vi "Data Viewer.vi"(6 "menu options":cluster{"open":bool, "save":bool, "view":bool}={"open"=TRUE, "save"=FALSE, "view"=FALSE}, 8 "error in (no error)":errorcluster, 9 "Stop Pointer":refnum<class "Pointer.lvclass">, 10 "Framework Configuration":T1, 11 "DSF":refnum<class "Framework.lvclass">) -> (0 "error out":errorcluster)   [LabVIEW 2017, in "DSF Data Viewer.lvlib"]
uses:
  DSF Data Viewer.lvlib
  Builds/Data Sharing Framework/Current/Core/DSF Core.lvlibp/Engine/Classes/Framework/Framework.lvclass
  Builds/Data Sharing Framework/Current/Core/DSF Core.lvlibp/DSF Configuration API/Public/Controls/DSF Engine Framework Configuration.ctl
  Builds/Data Sharing Framework/Current/Core/DSF Core.lvlibp/DSF Configuration API/Public/Controls/DSF Engine Plugin Configuration.ctl
  Builds/Data Sharing Framework/Current/Core/DSF Core.lvlibp/DSF Configuration API/Public/Controls/DSF Timing Info.ctl
  Builds/Data Sharing Framework/Current/Core/DSF Core.lvlibp/DSF Configuration API/Public/Controls/DSF Engine Plugin Thread Configuration.ctl
  Builds/Data Sharing Framework/Current/Core/DSF Core.lvlibp/DSF Configuration API/Public/Controls/DSF Settings Info.ctl
  Builds/Data Sharing Framework/Current/Core/DSF Core.lvlibp/DSF Configuration API/Public/Controls/DSF Engine Transfer Group Configuration.ctl
  Builds/Data Sharing Framework/Current/Core/DSF Core.lvlibp/DSF Configuration API/Public/Controls/DSF Direction.ctl
  Builds/Data Sharing Framework/Current/Core/DSF Core.lvlibp/DSF Configuration API/Public/Controls/DSF Engine Transfer Configuration.ctl
  Builds/Data Sharing Framework/Current/Core/DSF Core.lvlibp/DSF Configuration API/Public/Controls/DSF Byte Order.ctl
  Builds/Data Sharing Framework/Current/Core/DSF Core.lvlibp/DSF Configuration API/Public/Controls/DSF Engine Channel Configuration.ctl
  Builds/Data Sharing Framework/Current/Core/DSF Core.lvlibp/DSF Configuration API/Public/Controls/DSF Data Type.ctl
  Builds/Data Sharing Framework/Current/Core/DSF Core.lvlibp/DSF Configuration API/Public/Controls/DSF Timeout Behavior.ctl
  <vilib>/NI/Memory Manager/Classes/Pointer/Pointer.lvclass
  <vilib>/NI/Memory Manager/Classes/Pointer/Pointer.lvclass/Pointer.ctl
  Source/Main VI/Application Data.ctl
  Source/Buffer Reader/Buffer Data.ctl
  Builds/Data Sharing Framework/Current/Core/DSF Core.lvlibp/Engine/Classes/Buffer/Buffer.lvclass
  Builds/Data Sharing Framework/Current/Core/DSF Core.lvlibp/Engine/Classes/Transfer Group Status/Transfer Group Status.lvclass
  <vilib>/NI/Memory Manager/Classes/Pointer/Read Bool.vi
  <vilib>/NI/Memory Manager/Classes/Pointer/Write Bool.vi
  <vilib>/NI/Memory Manager/Classes/Pointer/Read (No Check).vi
  <vilib>/NI/Memory Manager/Classes/Pointer/Read (No Check) Bool.vi
  <vilib>/NI/Memory Manager/Classes/Pointer/Check Move.vi
  <vilib>/NI/Memory Manager/Classes/Pointer/Write (No Check).vi
  <vilib>/NI/Memory Manager/Classes/Pointer/Write (No Check) Bool.vi
  <vilib>/NI/Memory Manager/Classes/Pointer/Get Address.vi
  <vilib>/NI/Memory Manager/Classes/Pointer/Set Address.vi
  <vilib>/NI/Memory Manager/Classes/Pointer/Set Size.vi
  <vilib>/NI/Memory Manager/Classes/Pointer/Set Internal.vi
  <vilib>/NI/Memory Manager/Classes/Pointer/Check Null Pointer.vi
  <vilib>/NI/Memory Manager/Classes/Pointer/Check Count.vi
  <vilib>/NI/Memory Manager/Classes/Pointer/Check Bounds (Power of 2).vi
  <vilib>/NI/Memory Manager/Classes/Pointer/Errors.vi
  <vilib>/NI/Memory Manager/Classes/Pointer/Null Pointer.vi
  <vilib>/NI/Memory Manager/Classes/Pointer/Get Size.vi
  <vilib>/NI/Memory Manager/Classes/Pointer/Out of Bounds.vi
  <vilib>/NI/Memory Manager/Classes/Pointer/Check Bounds.vi
  <vilib>/NI/Memory Manager/Classes/Pointer/Create Error.vi
  <vilib>/NI/Memory Manager/VIs/Source.Write.String.vi
  <vilib>/NI/Memory Manager/Classes/Pointer/Write Pointer Size.vi
  <vilib>/NI/Memory Manager/VIs/Source.Write.Scalar.Base10.vi
  <vilib>/NI/Memory Manager/VIs/Source.Write.Scalar.Base10 (U64).vi
  <vilib>/NI/Memory Manager/Classes/Pointer/Check Pointer Bounds.vi
  <vilib>/NI/Memory Manager/Classes/Pointer/Check Buffer Bounds.vi
  <vilib>/NI/Memory Manager/VIs/New Error Cluster Constant.vi
  <vilib>/NI/Memory Manager/VIs/New Error Cluster Constant (512B).vi
  <vilib>/NI/Memory Manager/VIs/Error Cluster.Set Status.vi
  <vilib>/NI/Memory Manager/VIs/Error Cluster.Set Code.vi
  <vilib>/NI/Memory Manager/VIs/Error Cluster.Set VI Source.vi
  <vilib>/NI/Memory Manager/Constants/Constants.vi
  <vilib>/NI/Memory Manager/Constants/Library Name.vi
  <vilib>/NI/Memory Manager/Classes/Pointer/Pointer Error Info.vi
  <vilib>/NI/Memory Manager/Constants/Pointer Class Name.vi
  <vilib>/NI/Memory Manager/Classes/Pointer/Buffer Underflow.vi
  Builds/Data Sharing Framework/Current/Core/DSF Core.lvlibp/DSF Configuration API/Public/Largest Buffer Size (Framework).vi
  Builds/Data Sharing Framework/Current/Core/DSF Core.lvlibp
  Builds/Data Sharing Framework/Current/Core/DSF Core.lvlibp/Engine/Classes/Status/Performance.lvclass
panel:
  in  "Item Tree":string(tree)
  out "Late Count":u64
  out "Iteration":u64
  out "Frequency":dbl format="%.1fHz"
  out "Size":u64 format="%#_3pB"
  out "Null":bool
  out "Decimation":u64
  out "Throughput":dbl format="%#_3pBps"
  out "Buffer":string
  # "Data Viewer"
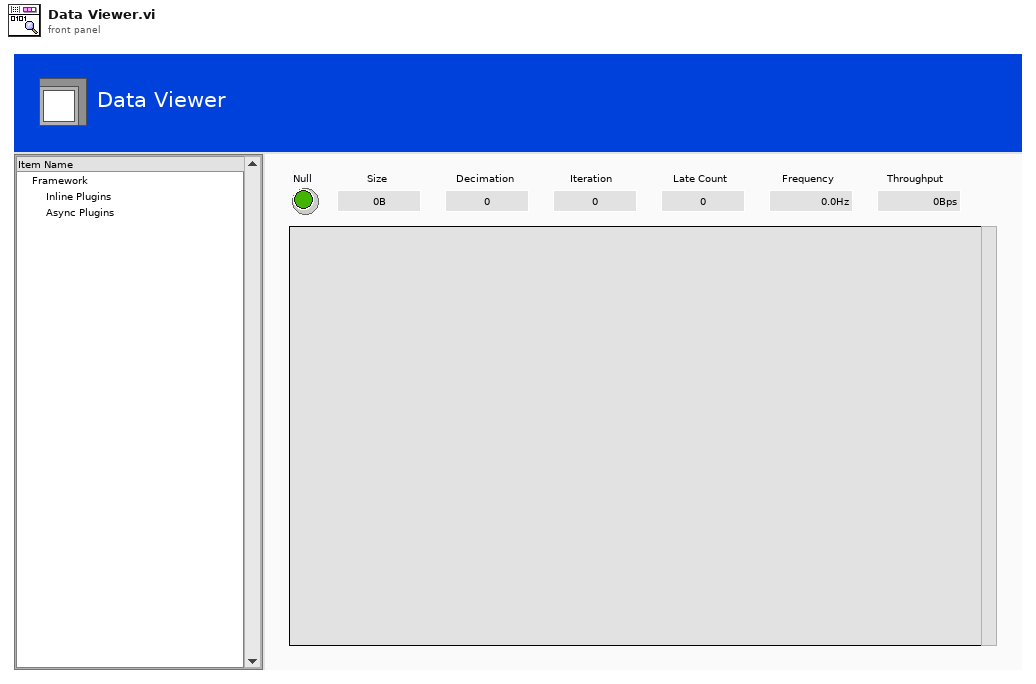
[diagram p1: front panel]
types:
  T1 = typedef "DSF Core.lvlibp/DSF Engine Framework Configuration.ctl" = cluster{"components directory":path, "Plugins":T2[]}
  T2 = typedef "DSF Core.lvlibp/DSF Engine Plugin Configuration.ctl" = cluster{"name":string, "components":string[], "cycle timing":T3, "threads":T4[], "Transfer Groups":T6[], "settings":T5}
  T3 = typedef "DSF Core.lvlibp/DSF Timing Info.ctl" = cluster{"priority":u64, "decimation":u64, "offset":u64}
  T4 = typedef "DSF Core.lvlibp/DSF Engine Plugin Thread Configuration.ctl" = cluster{"buffer converter settings":T5, "transceiver settings":T5, "processor":i32, "priority offset":i16}
  T5 = typedef "DSF Core.lvlibp/DSF Settings Info.ctl" = cluster{"key":string, "value":string}[]
  T6 = typedef "DSF Core.lvlibp/DSF Engine Transfer Group Configuration.ctl" = cluster{"name":string, "direction":T7, "cycle timing":T3, "thread index":i32, "settings":T5, "Transfers":T8[], "timeout behavior":T12}
  T7 = typedef "DSF Core.lvlibp/DSF Direction.ctl" = enum8{"Tx", "Rx"}
  T8 = typedef "DSF Core.lvlibp/DSF Engine Transfer Configuration.ctl" = cluster{"name":string, "byte order":T9, "settings":T5, "channels":T10[]}
  T9 = typedef "DSF Core.lvlibp/DSF Byte Order.ctl" = enum8{"big-endian", "little-endian"}
  T10 = typedef "DSF Core.lvlibp/DSF Engine Channel Configuration.ctl" = cluster{"string offset":u64, "string data type":T11, "engine data type":T11, "name":string, "settings":T5}
  T11 = typedef "DSF Core.lvlibp/DSF Data Type.ctl" = enum8{"Bool", "SGL", "DBL", "I8", "I16", "I32", "I64", "U8", "U16", "U32", "U64"}
  T12 = typedef "DSF Core.lvlibp/DSF Timeout Behavior.ctl" = enum8{"Increment Late Count", "Throw Error"}
  T13 = typedef "DSF Data Viewer.lvlib/Buffer Data.ctl" = cluster{"DSF Core.lvlibp:Buffer":refnum<class "Buffer.lvclass">, "DSF Core.lvlibp:Transfer Group Status.lvclass":refnum<class "Transfer Group Status.lvclass">, "decimation":u64}
  T14 = typedef "DSF Data Viewer.lvlib/Application Data.ctl" = cluster{"Item Tree Control":refnum<vi>, "Top-Level VI":refnum<vi>, "menu reference":refnum<k9>, "DSF Core.lvlibp:Framework":refnum<class "Framework.lvclass">, "buffer queue":refnum<queue>, "Stop Pointer":refnum<class "Pointer.lvclass">, "Buffer Variant":variant}
  T15 = typedef "DSF Core.lvlibp/DSF Transfer Group Status.ctl" = cluster{"late count":u64, "iteration":u64}
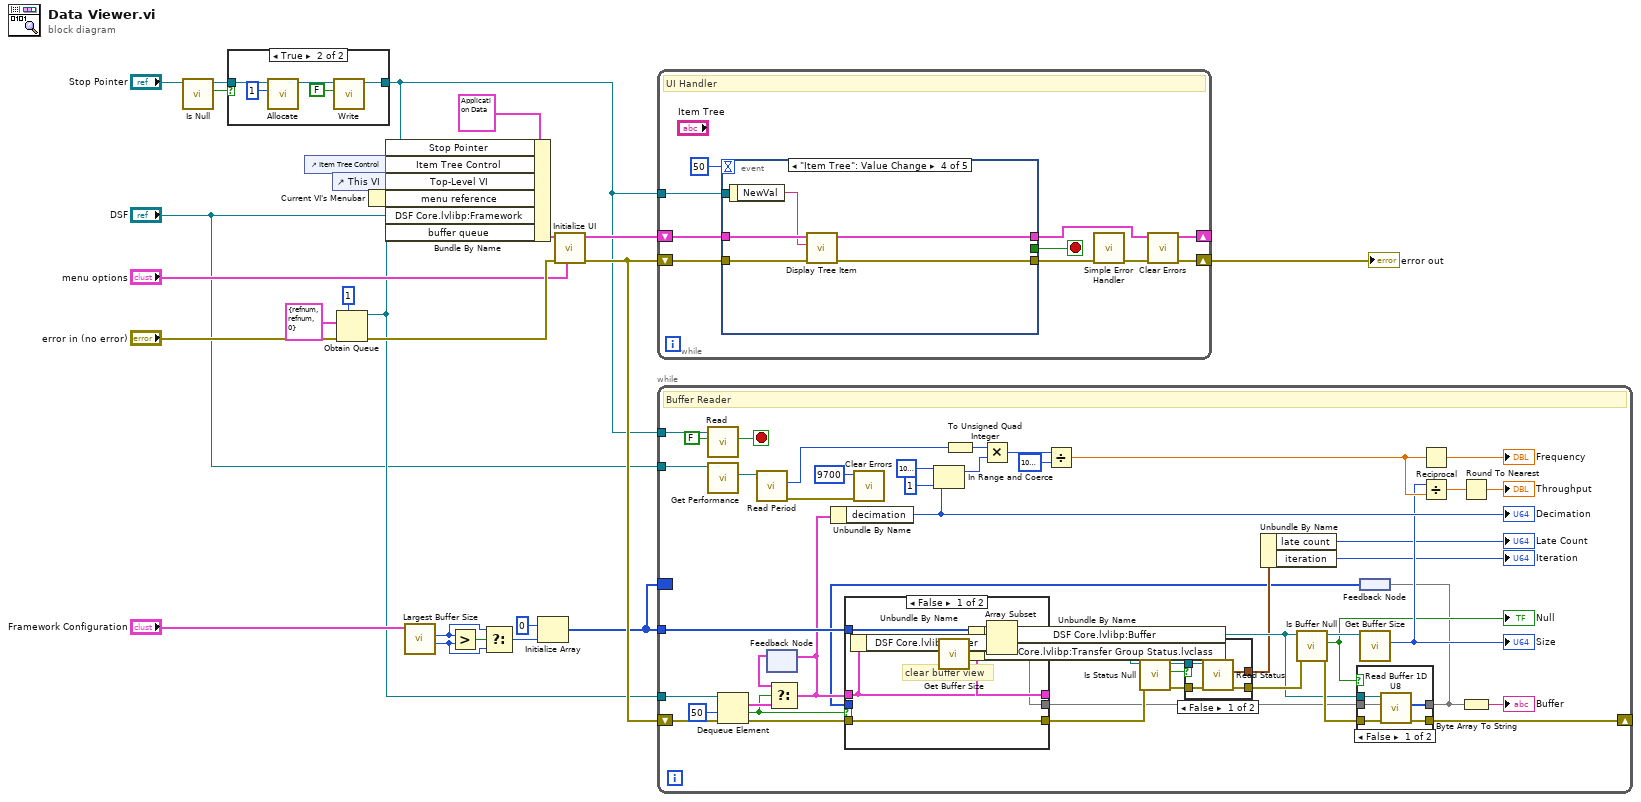
[diagram p0: block diagram]
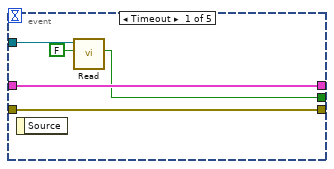
[diagram p6: hidden frame]
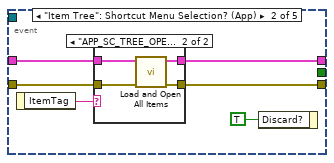
[diagram p7: hidden frame]
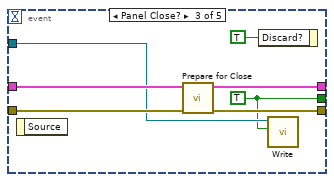
[diagram p9: hidden frame]
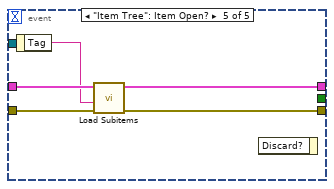
[diagram p10: hidden frame]
diagram:
  n1 = call <vilib>:"Is Null.vi"("Pointer in"="Stop Pointer") -> ("null?"=w6:bool)  [unwired: 8 in, 2 out]
  n2 = case shown="True" w6 {
    tunnel: [w26 w28] -> w4
    tunnel: "Stop Pointer" -> [w26 w30]
    frame False {
    }
    frame True {
      n3 = call <vilib>:"Allocate.vi"("size"=u64 1, "Pointer in"=w30) -> ("Pointer out"=w29:refnum<class "Pointer.lvclass">)  [unwired: 8 in, 1 out]
      n4 = call-poly <vilib>:"Write.vi"("value"=FALSE ("buffer in"), "Pointer in"=w29) -> ("Pointer out"=w28:refnum<class "Pointer.lvclass">)  [unwired: 6 in, 3 out]
    }
  }
  n5 = control-ref of="Item Tree Control"() -> (w21:refnum<vi>)
  n6 = control-ref of="This VI"() -> (w24:refnum<vi>)
  n7 = Obtain Queue(max queue size (-1, unlimited)=1, element data type=T13 {"DSF Core.lvlibp:Buffer"=refnum, "DSF Core.lvlibp:Transfer Group Status.lvclass"=refnum, "decimation"=0} ("Buffer data"), error in (no error)="error in (no error)") -> (queue out=w3:refnum<queue>, error out=w17:errorcluster)  [unwired: 2 in, 1 out]
  n8 = Current VI's Menubar() -> (w22:refnum<k9>)
  n9 = Bundle By Name(cluster=T14 {"Item Tree Control"=refnum, "Top-Level VI"=refnum, "menu reference"=refnum, "DSF Core.lvlibp:Framework"=refnum, "buffer queue"=refnum, "Stop Pointer"=refnum, "Buffer Variant"=variant}, "Stop Pointer"=w4, "Item Tree Control"=w21, "Top-Level VI"=w24, "menu reference"=w22, "DSF Core.lvlibp:Framework"="DSF", "buffer queue"=w3) -> (w20:T14)
  n10 = call-poly "Largest Buffer Size.vi"("Framework Configuration in"="Framework Configuration") -> ("largest engine buffer size"=w13:u64, "largest string buffer size"=w14:u64)  [unwired: 7 in, 2 out]
  n11 = Greater?(x=w14, y=w13) -> (0:w15:bool)
  n12 = Select(t=w14, s=w15, f=w13) -> (s? t:f=w11:u64)
  n13 = Initialize Array(u8 0 ("element"), w11) -> (w1:u8[])
  n14 = call "Initialize UI.vi"("menu options"="menu options", "error in (no error)"=w17, "Application Data in"=w20) -> ("error out"=w5:errorcluster, "Application Data out"=w9:T14)  [unwired: 7 in]
  n15 = while {
    shift-right: [w36] -> w23
    shift-left: w5 -> [w40]
    shift-right: [w37] -> _
    shift-left: w9 -> [w35]
    tunnel: w4 -> [w33]
    stop <- w34 stop-if-true
    # "UI Handler"
    n16 = event shown="[3] \"Item Tree\": Value Change" {
      selector: _ -> [_ _ _ _ _]
      dyn-events: _ -> [_ _ _ _ _]
      timeout: 50 -> [_ _ _ _ _]
      tunnel: [w41 _ w58 _ _] -> w34
      tunnel: w40 -> [w45 w48 w64 w69 w74]
      tunnel: [w45 w49 w62 w68 w73] -> w38
      tunnel: w35 -> [w44 w50 w60 w66 w72]
      tunnel: [w44 w46 w61 w67 w71] -> w37
      tunnel: w33 -> [w43 _ w59 _ _]
      event Timeout {
        n17 = event-data() -> ()  [unwired: 1 in, 1 out]
        n18 = call-poly <vilib>:"Read.vi"("value in"=FALSE ("buffer in"), "Pointer in"=w43) -> ("value out"=w41:bool)  [unwired: 6 in, 3 out]
      }
      event "Item Tree": Shortcut Menu Selection? (App) {
        n19 = event-data() -> ("ItemTag"=w51:string)  [unwired: 1 in]
        n20 = case shown="\"APP_SC_TREE_OPEN_ALL_ITEMS\"" w51 {
          tunnel: w50 -> [w52 w57]
          tunnel: [w53 w55] -> w49
          tunnel: w48 -> [w53 w56]
          tunnel: [w52 w54] -> w46
          frame Default {
          }
          frame "APP_SC_TREE_OPEN_ALL_ITEMS" {
            n21 = call "Load and Open All Items.vi"("error in (no error)"=w56, "Application Data in"=w57) -> ("error out"=w55:errorcluster, "Application Data out"=w54:T14)  [unwired: 8 in]
          }
        }
        n22 = event-data("Discard?"=TRUE) -> ()  [unwired: 1 in, 1 out]
      }
      event Panel Close? {
        w58 = TRUE
        n23 = event-data() -> ()  [unwired: 1 in, 1 out]
        n24 = call "Prepare for Close.vi"("error in (no error)"=w64, "Application Data in"=w60) -> ("error out"=w62:errorcluster, "Application Data out"=w61:T14)  [unwired: 8 in]
        n25 = event-data("Discard?"=TRUE) -> ()  [unwired: 1 in, 1 out]
        n26 = call-poly <vilib>:"Write.vi"("value"=w58, "Pointer in"=w59) -> ()  [unwired: 6 in, 4 out]
      }
      event "Item Tree": Value Change {
        n27 = event-data() -> ("NewVal"=w65:string)  [unwired: 1 in]
        n28 = call "Display Tree Item.vi"("error in (no error)"=w69, "Tag"=w65, "Application Data in"=w66) -> ("error out"=w68:errorcluster, "Application Data out"=w67:T14)  [unwired: 7 in]
      }
      event "Item Tree": Item Open? {
        n29 = event-data() -> ("Tag"=w70:string)  [unwired: 1 in]
        n30 = call "Load Subitems.vi"("error in (no error)"=w74, "Tag"=w70, "Application Data in"=w72) -> ("error out"=w73:errorcluster, "Application Data out"=w71:T14)  [unwired: 6 in, 1 out]
        n31 = event-data() -> ()  [unwired: 2 in, 1 out]
      }
    }
    n32 = call <vilib>:"Simple Error Handler.vi"("error in (no error)"=w38) -> ("error out"=w39:errorcluster)  [unwired: 4 in, 4 out]
    n33 = call <vilib>:"Clear Errors.vi"("error in (no error)"=w39) -> ("error out"=w36:errorcluster)  [unwired: 5 in, 1 out]
  }
  "error out" <- w23
  n34 = while {
    tunnel: w3 -> [w121]
    shift-right: [w93] -> _
    shift-left: w5 -> [w118]
    tunnel: w1 -> [w108]
    tunnel: w4 -> [w112]
    tunnel: "DSF" -> [w105]
    border: w1 -> [_]
    stop <- w113 stop-if-true
    # "Buffer Reader"
    n35 = call-poly <vilib>:"Read.vi"("value in"=FALSE ("buffer in"), "Pointer in"=w112) -> ("value out"=w113:bool)  [unwired: 6 in, 3 out]
    n36 = call "Get Performance.vi"("Framework in"=w105) -> ("Performance"=w104:refnum<class "Performance.lvclass">)  [unwired: 9 in, 1 out]
    n37 = Dequeue Element(queue=w121, timeout in ms (-1)=50, error in (no error)=w118) -> (element=w119:T13, timed out?=w109:bool, error out=w122:errorcluster)  [unwired: 1 out]
    n38 = call "Read Period.vi"("Framework Performance in"=w104) -> ("error out"=w94:errorcluster, "period"=w102:u32)  [unwired: 8 in, 1 out]
    n39 = feedback #1() -> (w107:T13)  [unwired: 1 in]
    n40 = Select(t=w107, s=w109, f=w119) -> (s? t:f=w97:T13)
    n41 = feedback-in #1(w97) -> ()
    n42 = Unbundle By Name(w97) -> ("decimation"=w98:u64)
    "Decimation" <- w98
    n43 = call <vilib>:"Clear Errors.vi"("error in (no error)"=w94, "specific error code to clear (0: all)"=9700) -> ()  [unwired: 4 in, 2 out]
    n44 = In Range and Coerce(upper limit=u64 1000000000, x=w98, lower limit=u64 1) -> (coerced(x)=w99:u64)  [unwired: 1 out]
    n45 = To Unsigned Quad Integer(1:w102) -> (0:w101:u64)
    n46 = Multiply(x=w101, y=w99) -> (x*y=w117:u64)
    n47 = Divide(x=w117, y=u64 1000000) -> (x/y=w100:dbl)
    n48 = feedback #2() -> (w76:u8[])
    n49 = case shown="False" w109 {
      tunnel: w76 -> [_ w143]
      tunnel: w97 -> [w136 w142]
      tunnel: w108 -> [w140 _]
      tunnel: [w135 w143] -> w77
      tunnel: w122 -> [w137 w141]
      tunnel: [w136 w142] -> w103
      tunnel: [w137 w141] -> w84
      frame False {
        # "clear buffer view"
        n50 = Unbundle By Name(w136) -> ("DSF Core.lvlibp:Buffer"=w138:refnum<class "Buffer.lvclass">)
        n51 = call "Get Buffer Size.vi"("Buffer in"=w138) -> ("buffer size"=w139:u64)  [unwired: 9 in, 1 out]
        n52 = Array Subset(array=w140, length=w139) -> (w135:u8[])  [unwired: 1 in]
      }
      frame True {
      }
    }
    n53 = Unbundle By Name(w103) -> ("DSF Core.lvlibp:Buffer"=w88:refnum<class "Buffer.lvclass">, "DSF Core.lvlibp:Transfer Group Status.lvclass"=w87:refnum<class "Transfer Group Status.lvclass">)
    n54 = call "Is Status Null.vi"("error in (no error)"=w84, "Transfer Group Status in"=w87) -> ("error out"=w85:errorcluster, "null?"=w83:bool, "Transfer Group Status out"=w86:refnum<class "Transfer Group Status.lvclass">)  [unwired: 7 in]
    n55 = case shown="False" w83 {
      tunnel: [w126 w127] -> w89
      tunnel: w86 -> [w125 _]
      tunnel: w85 -> [w124 w127]
      tunnel: [w123 _] -> w82
      frame False {
        n56 = call "Read Status.vi"("error in (no error)"=w124, "Transfer Group Status in"=w125) -> ("error out"=w126:errorcluster, "status"=w123:T15)  [unwired: 7 in, 1 out]
      }
      frame True {
      }
    }
    n57 = Unbundle By Name(w82) -> ("late count"=→"Late Count":u64, "iteration"=→"Iteration":u64)
    n58 = call "Is Buffer Null.vi"("error in (no error)"=w89, "Buffer in"=w88) -> ("error out"=w91:errorcluster, "null?"=w90:bool, "Buffer out"=w92:refnum<class "Buffer.lvclass">)  [unwired: 7 in]
    "Null" <- w90
    n59 = case shown="False" w90 {
      tunnel: w91 -> [w132 w133]
      tunnel: w77 -> [w131 w134]
      tunnel: w88 -> [w130 _]
      tunnel: [w129 w134] -> w79
      tunnel: [w128 w133] -> w93
      frame False {
        n60 = call "Read Buffer 1D U8.vi"("error in (no error)"=w132, "dst array in"=w131, "Buffer in"=w130) -> ("error out"=w128:errorcluster, "dst array out"=w129:u8[])  [unwired: 5 in, 2 out]
      }
      frame True {
      }
    }
    n61 = feedback-in #2(w79) -> ()
    n62 = call "Get Buffer Size.vi"("Buffer in"=w92) -> ("buffer size"=w96:u64)  [unwired: 9 in, 1 out]
    "Size" <- w96
    n63 = Reciprocal(x=w100) -> (1/x=→"Frequency":dbl)
    n64 = Divide(x=w96, y=w100) -> (x/y=w115:dbl)
    n65 = Round To Nearest(number=w115) -> (nearest integer value=→"Throughput":dbl)
    n66 = Byte Array To String(unsigned byte array=w79) -> (string=→"Buffer":string)
  }
